vi "myRIO_BRig_Host_parse_dataTrial__readMain__v2.vi"(0 "input_idxUnknown":i32, 1 "input_arrayUnknown":i32[][](array[numeric]), 2 "input_idxReward":i32, 3 "input_arrayReward":i32[][](array[numeric]), 4 "input_idxWrong":i32, 5 "input_arrayWrong":i32[][](array[numeric]), 6 "input_idxTimeout":i32, 7 "input_arrayTimeout":i32[][](array[numeric]), 10 "arrayIn_dataTrial":u16[][](array[numeric]), 12 "arrayIn_empty":i32[][](array[numeric])) -> (20 "output_idxUnknown":i32, 21 "output_arrayUnknown":i32[][](array[numeric]), 22 "output_idxReward":i32, 23 "output_arrayReward":i32[][](array[numeric]), 24 "output_idxWrong":i32, 25 "output_arrayWrong":i32[][](array[numeric]), 26 "output_idxTimeout":i32, 27 "output_arrayTimeout":i32[][](array[numeric]))   [LabVIEW 2014]
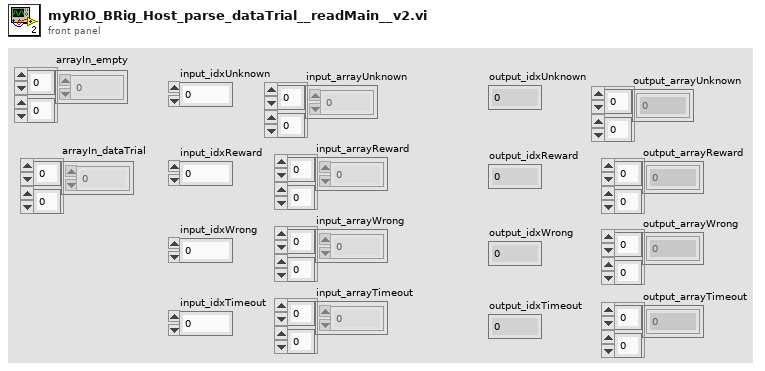
[diagram p1: front panel]
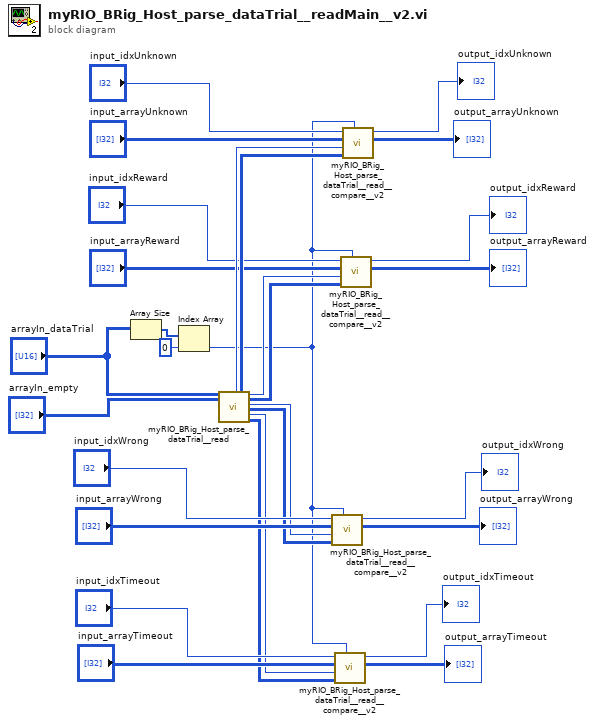
[diagram p0: block diagram]
diagram:
  n1 = Array Size(array="arrayIn_dataTrial") -> (size(s)=w4:i32[])
  n2 = Index Array(array=w4, index=0) -> (element=w1:i32)
  n3 = call "myRIO_BRig_Host_parse_dataTrial__read.vi"("arrayIn_dataTrial"="arrayIn_dataTrial", "arrayIn_empty"="arrayIn_empty") -> ("output_idxUnknown"=w26:i32, "output_arrayUnknown"=w25:i32[][], "output_idxReward"=w22:i32, "output_arrayReward"=w21:i32[][], "output_idxWrong"=w18:i32, "output_arrayWrong"=w17:i32[][], "output_idxTimeout"=w14:i32, "output_arrayTimeout"=w13:i32[][])  [unwired: 10 in]
  n4 = call "myRIO_BRig_Host_parse_dataTrial__read__compare__v2.vi"("input_maxTrials_Ctrl"=w1, "input_arrayCtrl"=w17, "input_idxCtrl"=w18, "input_arraySample"="input_arrayWrong", "input_idxSample"="input_idxWrong") -> ("output_arraySample"=→"output_arrayWrong":i32[][], "output_idxSample"=→"output_idxWrong":i32)  [unwired: 5 in]
  n5 = call "myRIO_BRig_Host_parse_dataTrial__read__compare__v2.vi"("input_maxTrials_Ctrl"=w1, "input_arrayCtrl"=w13, "input_idxCtrl"=w14, "input_arraySample"="input_arrayTimeout", "input_idxSample"="input_idxTimeout") -> ("output_arraySample"=→"output_arrayTimeout":i32[][], "output_idxSample"=→"output_idxTimeout":i32)  [unwired: 5 in]
  n6 = call "myRIO_BRig_Host_parse_dataTrial__read__compare__v2.vi"("input_maxTrials_Ctrl"=w1, "input_arrayCtrl"=w21, "input_idxCtrl"=w22, "input_arraySample"="input_arrayReward", "input_idxSample"="input_idxReward") -> ("output_arraySample"=→"output_arrayReward":i32[][], "output_idxSample"=→"output_idxReward":i32)  [unwired: 5 in]
  n7 = call "myRIO_BRig_Host_parse_dataTrial__read__compare__v2.vi"("input_maxTrials_Ctrl"=w1, "input_arrayCtrl"=w25, "input_idxCtrl"=w26, "input_arraySample"="input_arrayUnknown", "input_idxSample"="input_idxUnknown") -> ("output_arraySample"=→"output_arrayUnknown":i32[][], "output_idxSample"=→"output_idxUnknown":i32)  [unwired: 5 in]
